vi "Trap1-24-03-2017.vi"(0 "Periode(us)":u32, 1 "zwischenMesswerten(us)":u16, 2 "Warten(us)":u16, 5 "5Van(us)":u16, 7 "Heizen":bool, 9 "Messwerte":i32, 11 "setpoint":fxp<+/-,16,6> format="%.12g", 12 "PID gains":T1={"proportional gain (Kc)"=1.0, "integral gain (Kc*Ts/Ti)"=1.66796875, "derivative gain (Kc*Td/Ts)"=0.0} {"proportional gain (Kc)" format="%.11g"; "integral gain (Kc*Ts/Ti)" format="%.11g"; "derivative gain (Kc*Td/Ts)" format="%.11g"}) -> (4 "Messwert":fxp<+/-,27,6> format="%.23g")   [LabVIEW 2010]
uses:
  <vilib>/eio/EIONode/EIONode.xnode
  <vilib>/rvi/eio/nirviEIOImplementation/nirviEIOImplementation.xnode
  <vilib>/rvi/eio/common/nirviEmuClasses.ctl
  <vilib>/rvi/FXPMathLib/FxpDiv/XNode/nifxpmath_Div.xnode
  <vilib>/rvi/FXPMathLib/FxpDiv/subVIs/nifxpmath_Div_SimConfig.ctl
  <vilib>/rvi/FXPMathLib/FxpAdd/XNode/nifxpmath_Add.xnode
  <vilib>/rvi/FXPMathLib/FxpAdd/subVIs/nifxpmath_Add_SimConfig.ctl
  <vilib>/fxp/LVFixedPointQuantizationPolicyTypeDef.ctl
  <vilib>/fxp/LVFixedPointOverflowPolicyTypeDef.ctl
  <vilib>/rvi/FXPMathLib/FxpConvert/XNode/nifxpmath_Convert.xnode
  <vilib>/rvi/FXPMathLib/FxpConvert/subVIs/nifxpmath_Convert_SimConfig.ctl
  <vilib>/addons/control/pid/fpga.llb/XNode/niFpgaPID.xnode
  <vilib>/rvi/FXPMathLib/FxpMul/XNode/nifxpmath_Multiplier.xnode
  <vilib>/rvi/FXPMathLib/FxpMul/subVIs/nifxpmath_Mul_SimConfig.ctl
  <vilib>/rvi/eio/common/nirviEmuTemplateMethod_noerrors.vi
  <vilib>/rvi/FXPMathLib/FxpDiv/simVIs/DllFxpDivTemp_sub.vi
  <vilib>/rvi/FXPMathLib/FxpAdd/simVIs/DllFxpAddTemp_sub.vi
  <vilib>/rvi/FXPMathLib/FxpConvert/simVIs/DllFxpConvertTemp_sub.vi
  <vilib>/rvi/FXPMathLib/FxpMul/simVIs/DllFxpMulTemp_sub.vi
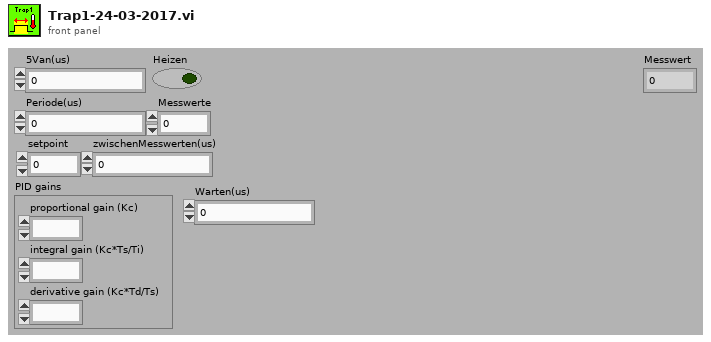
[diagram p1: front panel]
types:
  T1 = cluster{"proportional gain (Kc)":fxp<+/-,16,8>, "integral gain (Kc*Ts/Ti)":fxp<+/-,16,8>, "derivative gain (Kc*Td/Ts)":fxp<+/-,16,8>}
  T2 = typedef "nirviEmuClasses.ctl" = enum16{"IO Read", "IO Write", "Method", "Property Read", "Property Write"}
  T3 = cluster{"output high":fxp<+/-,16,6>, "output low":fxp<+/-,16,6>}
  T4 = cluster{"proportional gain (Kc)":i16, "integral gain (Kc*Ts/Ti)":i16, "derivative gain (Kc*Td/Ts)":i16}
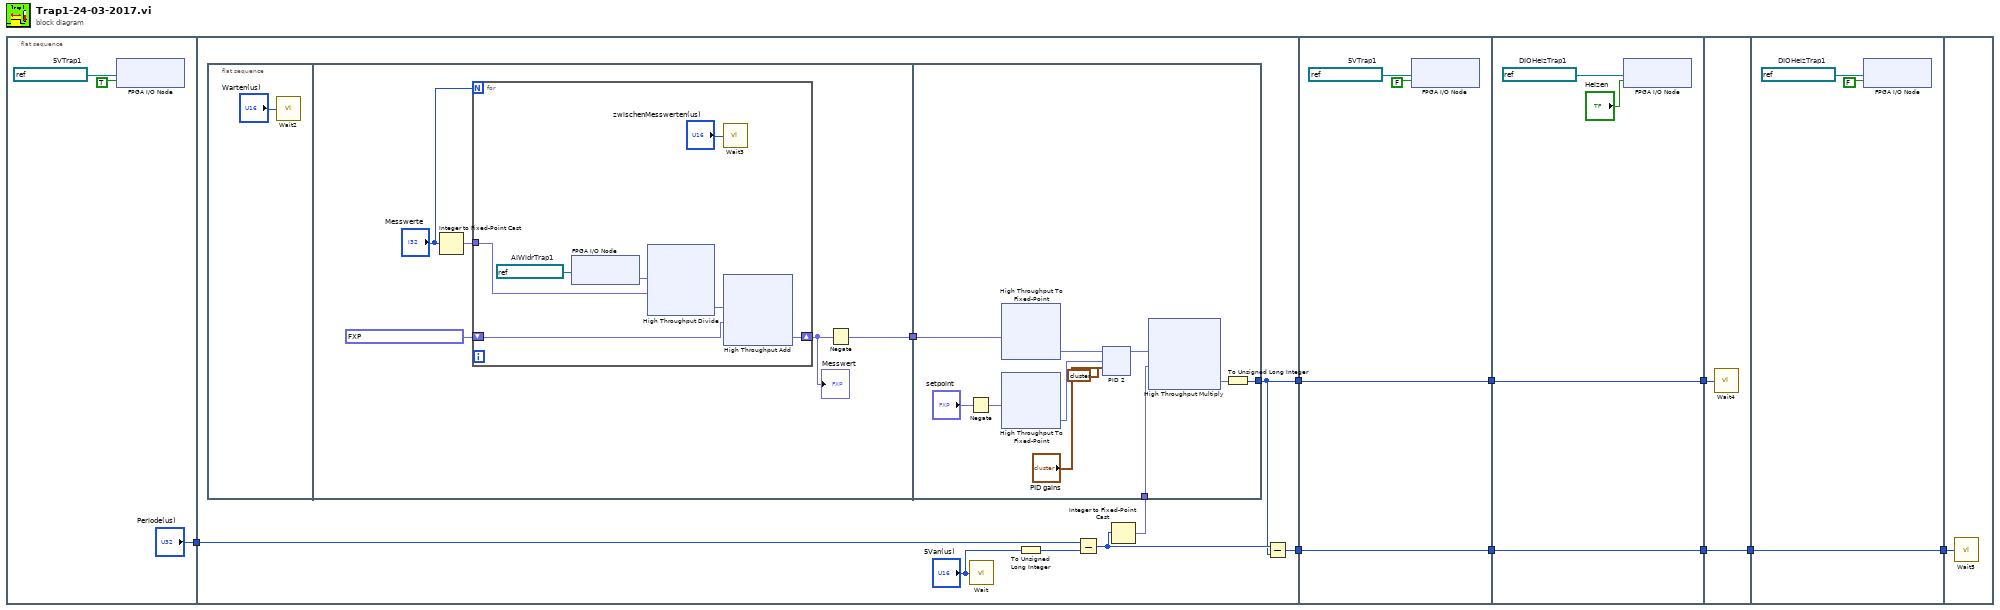
[diagram p0: block diagram]
diagram:
  n1 = flat-sequence {
    tunnel: ["Periode(us)"] -> w9
    tunnel: w9 -> [w30]
    tunnel: [w25] -> w7
    tunnel: [w24] -> w1
    tunnel: [w243] -> w8
    tunnel: w7 -> [w243]
    tunnel: [w242] -> w2
    tunnel: w1 -> [w242]
    tunnel: w8 -> [w258]
    tunnel: [w258] -> w6
    tunnel: [w257] -> w3
    tunnel: w2 -> [w257]
    tunnel: w6 -> [w273]
    tunnel: [w272] -> w4
    tunnel: w3 -> [w272]
    tunnel: [w274] -> w5
    tunnel: w4 -> [w274]
    tunnel: w5 -> [w288]
    frame #0 {
      w12 = refnum<k21> "Mod6/DIO21"  # 5VTrap1
      n2 = xnode "FPGA I/O Node"("I/O Item"=TRUE, "FPGA I/O In"=w12) -> ()  [unwired: 1 out]
    }
    frame #1 {
      n3 = flat-sequence {
        tunnel: [w35] -> w31
        tunnel: w31 -> [w131]
        tunnel: w27 -> [w126]
        tunnel: [w124] -> w25
        frame #0 {
          n4 = call "Wait2"("Count(uSec)"="Warten(us)") -> ()  [unwired: 1 out]
        }
        frame #1 {
          n5 = Integer to Fixed-Point Cast(integer="Messwerte") -> (fixed-point=w36:fxp<+/-,32,32>)  [unwired: 1 in]
          n6 = for {
            N: "Messwerte" -> [_]
            shift-right: [w40] -> w34
            shift-left: fxp<+/-,26,5> 0.0 ("I/O Item") -> [w41]
            tunnel: w36 -> [w38]
            w44 = refnum<k21> "Mod1/AI30"  # AIWidrTrap1
            n7 = xnode "FPGA I/O Node"("FPGA I/O In"=w44) -> ("I/O Item"=w43:fxp<+/-,26,5>)  [unwired: 1 out]
            n8 = xnode "High Throughput Divide"("x"=w43, "y"=w38) -> ("x/y"=w42:fxp<+/-,26,5>)
            n9 = call "Wait3"("Count(uSec)"="zwischenMesswerten(us)") -> ()  [unwired: 1 out]
            n10 = xnode "High Throughput Add"("x"=w42, "y"=w41) -> ("x+y"=w40:fxp<+/-,27,6>)
          }
          "Messwert" <- w34
          n11 = Negate(x=w34) -> (-x=w35:fxp<+/-,28,7>)
        }
        frame #2 {
          n12 = Negate(x="setpoint") -> (-x=w122:fxp<+/-,17,7>)
          n13 = xnode "High Throughput To Fixed-Point"("x"=w131) -> ("y"=w130:fxp<+/-,16,6>)
          n14 = xnode "High Throughput To Fixed-Point"("x"=w122) -> ("y"=w121:fxp<+/-,16,6>)
          n15 = xnode ("PID 2")("process variable"=w130, "setpoint"=w121, "PID gains"="PID gains", "output range"=T3 {"output high"=1.0, "output low"=0.0}) -> ("output"=w127:fxp<+/-,16,6>)  [unwired: 1 in]
          n16 = xnode "High Throughput Multiply"("x"=w127, "y"=w126) -> ("x*y"=w125:fxp<+/-,32,32>)
          n17 = To Unsigned Long Integer(number=w125) -> (unsigned 32bit integer=w124:u32)
        }
      }
      n18 = call "Wait"("Count(uSec)"="5Van(us)") -> ()  [unwired: 1 out]
      n19 = To Unsigned Long Integer(number="5Van(us)") -> (unsigned 32bit integer=w28:u32)
      n20 = Subtract(x=w30, y=w28) -> (x-y=w26:u32)
      n21 = Integer to Fixed-Point Cast(integer=w26) -> (fixed-point=w27:fxp<+,32,32>)  [unwired: 1 in]
      n22 = Subtract(x=w26, y=w25) -> (x-y=w24:u32)
    }
    frame #2 {
      w245 = refnum<k21> "Mod6/DIO21"  # 5VTrap1
      n23 = xnode "FPGA I/O Node"("I/O Item"=FALSE, "FPGA I/O In"=w245) -> ()  [unwired: 1 out]
    }
    frame #3 {
      w260 = refnum<k21> "Mod6/DIO19"  # DIOHeizTrap1
      n24 = xnode "FPGA I/O Node"("I/O Item"="Heizen", "FPGA I/O In"=w260) -> ()  [unwired: 1 out]
    }
    frame #4 {
      n25 = call "Wait4"("Count(uSec)"=w273) -> ()  [unwired: 1 out]
    }
    frame #5 {
      w276 = refnum<k21> "Mod6/DIO19"  # DIOHeizTrap1
      n26 = xnode "FPGA I/O Node"("I/O Item"=FALSE, "FPGA I/O In"=w276) -> ()  [unwired: 1 out]
    }
    frame #6 {
      n27 = call "Wait5"("Count(uSec)"=w288) -> ()  [unwired: 1 out]
    }
  }
